vi "FPGA move test 001.vi"() -> ()   [LabVIEW 2019]
uses:
  <vilib>/Platform/TimedLoop/XDataNode/timing_clust.ctl
  <vilib>/Platform/TimedLoop/XDataNode/nitl_modes.ctl
  <vilib>/Platform/TimedLoop/XDataNode/wakeup.ctl
  motor/motor single class/Motor single.lvclass
  motor/motor enum(FPGA).ctl
  motor/motor single class/Variable PID(Kp).ctl
  motor/motor single class/Variable PID(Kp) mode enum.ctl
  <vilib>/platform/TimedLoop/XDataNode/XDataNode.xnode
  <vilib>/Platform/TimedLoop/XDataNode/XDNodeRunTimeDep.lvlib
panel:
  in  "error in (no error)":errorcluster
  out "error out":errorcluster
  in  "RPM":dbl
  in  "Y":dbl
  in  "X":dbl
  out "out array":dbl[](array[numeric])
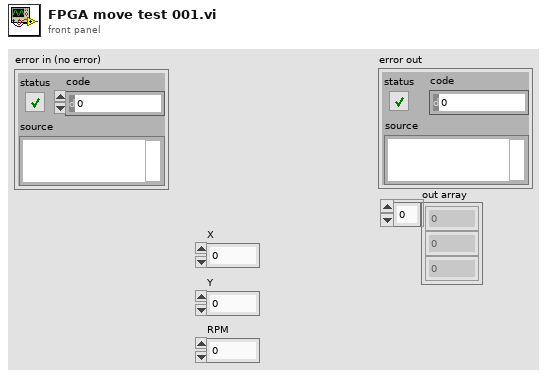
[diagram p1: front panel]
types:
  T1 = typedef "Motor single.lvclass/Variable PID(Kp).ctl" = cluster{"Enable variable PID(Kp)":bool, "Variable PID(Kp)range":dbl, "Variable MODE":T2}
  T2 = typedef "Motor single.lvclass/Variable PID(Kp) mode enum.ctl" = enum16{"Log", "Sin&Cos", "Linear", "reverse Log", "const"}
  T3 = typedef "Motor single.lvclass/motor enum(FPGA).ctl" = enum16{"M1", "M2", "M3", "M4"}
  T4 = typedef "XDNodeRunTimeDep.lvlib/timing_clust.ctl" = cluster{"Expected End [f-1]":u64, "Actual End [f-1]":u64, "Finished Late? [f-1]":bool, "Expected End [i-1]":u64, "Actual End [i-1]":u64, "Finished Late? [i-1]":bool, "Expected Start [i]":u64, "Actual Start [i]":u64, "Expected Start [f]":u64, "Actual Start [f]":u64, "Source Name":string, "Structure Name":string, "Period":i64, "Deadline":i64, "Offset":i64, "Start":i64, "Priority":i32, "Timeout":i32, "Mode":T5, "Wakeup Reason":T6, "Error":errorcluster, "Source Type":string, "Secondary Source Type":string, "Global End Time":u64, "Global Start Time":u64, "Frame Duration":u64, "Iteration Duration":u64, "Assigned CPU":i32, "I/O Scan Engine Mode":u32}
  T5 = typedef "XDNodeRunTimeDep.lvlib/nitl_modes.ctl" = enum32{"No Change", "Process missed periods, maintain original phase", "Discard missed periods, maintain original phase", "Process missed periods, ignore original phase", "Discard missed periods, ignore original phase"}
  T6 = typedef "XDNodeRunTimeDep.lvlib/wakeup.ctl" = enum32{"Normal", "Aborted", "Asynchronous wakeup", "Timing source error", "Timed loop error", "Timeout"}
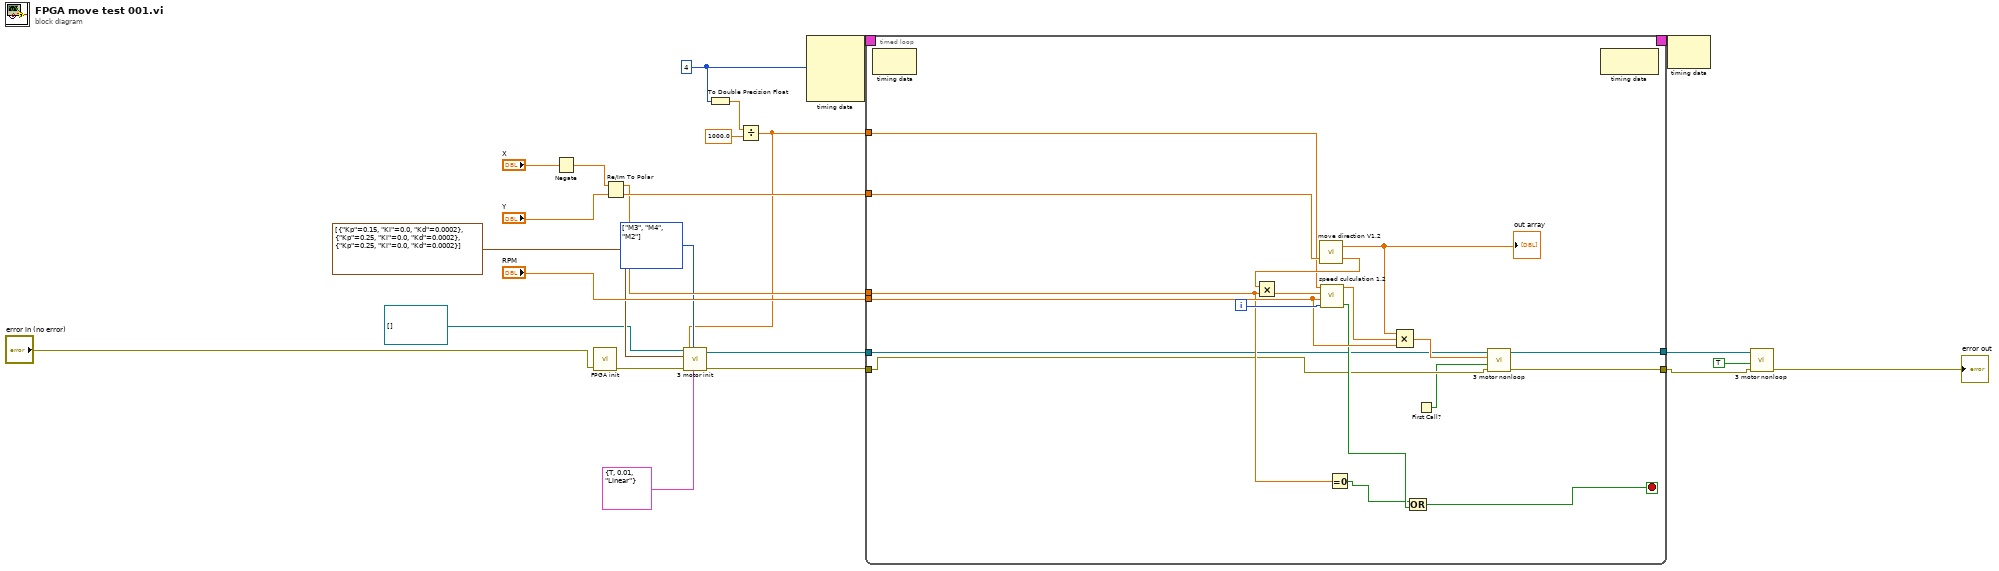
[diagram p0: block diagram]
diagram:
  w9 = T3[] [enum."M3", enum."M4", enum."M2"] items=["M1", "M2", "M3", "M4"] ("Array 2")
  w22 = i64 4 ("Period")
  n1 = Negate(x="X") -> (-x=w14:dbl)
  n2 = call "FPGA init.vi"("error in"="error in (no error)") -> ("error out"=w13:errorcluster)  [unwired: 9 in, 1 out]
  n3 = Re/Im To Polar(2:"Y", 3:w14) -> (0:w18:dbl, 1:w17:dbl)
  n4 = To Double Precision Float(number=w22) -> (double precision float=w21:dbl)
  n5 = Divide(x=w21, y=1000.0) -> (x/y=w6:dbl)
  n6 = call "3 motor init.vi"("Variable PID(Kp)"=T1 {"Enable variable PID(Kp)"=TRUE, "Variable PID(Kp)range"=0.01, "Variable MODE"=enum."Linear"}, "Array 2"=w9, "Error In"=w13, "dt(s)"=w6, "PID"=cluster{"Kp":dbl, "Ki":dbl, "Kd":dbl}[] [{"Kp"=0.15, "Ki"=0.0, "Kd"=0.0002}, {"Kp"=0.25, "Ki"=0.0, "Kd"=0.0002}, {"Kp"=0.25, "Ki"=0.0, "Kd"=0.0002}], "Array"=refnum<class "Motor single.lvclass">[] []) -> ("error out"=w7:errorcluster, "Object array"=w5:refnum<class "Motor single.lvclass">[])  [unwired: 4 in]
  n7 = node-c288(w22) -> (w24:T4)  [unwired: 3 in]
  n8 = timed-loop {
    timing: w24 -> [_]
    timing-out: [_] -> w23
    tunnel: w18 -> [w41]
    tunnel: w17 -> [w30]
    tunnel: "RPM" -> [w34]
    tunnel: w7 -> [w29]
    tunnel: [w39] -> w3
    tunnel: w6 -> [w28]
    tunnel: w5 -> [w27]
    tunnel: [w25] -> w1
    i -> [w42]
    stop <- w32 stop-if-true
    n9 = node-c288() -> ()  [unwired: 1 in, 1 out]
    n10 = call "move direction V1.2.vi"("theta"=w41) -> ("max value"=w35:dbl, "out array"=w40:dbl[])  [unwired: 1 in]
    "out array" <- w40
    n11 = Multiply(x=w35, y=w30) -> (x*y=w36:dbl)
    n12 = call "speed culculation 1.2.vi"("i"=w42, "Speed(RPM)"=w34, "distance"=w36, "dt(s)"=w28) -> ("complet?"=w33:bool, "Speed"=w37:dbl)  [unwired: 4 in, 2 out]
    n13 = Equal To 0?(x=w30) -> (x = 0?=w31:bool)
    n14 = Compound Arithmetic op=MULTIPLY(w40, w37, w34) -> (w38:dbl[])
    n15 = Compound Arithmetic op=OR(w31, w33) -> (w32:bool)
    n16 = First Call?() -> (First Call?: T/F=w26:bool)
    n17 = call "3 motor nonloop.vi"("Error In"=w29, "Reset"=w26, "speed"=w38, "Array"=w27) -> ("error out"=w39:errorcluster, "appended array"=w25:refnum<class "Motor single.lvclass">[])  [unwired: 3 in, 3 out]
    n18 = node-c288() -> ()  [unwired: 1 in, 1 out]
  }
  n19 = node-c288(w23) -> ()  [unwired: 1 out]
  n20 = call "3 motor nonloop.vi"("Error In"=w3, "Reset"=TRUE, "Array"=w1) -> ("error out"=→"error out":errorcluster)  [unwired: 4 in, 4 out]
